vi "Set dts in Channel Groups.vi"(8 "error in":errorcluster, 9 "channel groups decimations":dbl[](array[numeric]), 11 "File Log Spec in":T1 {"File Node Ref" format="%.0x"}) -> (0 "error out":errorcluster, 3 "File Log Spec out":T1 {"File Node Ref" format="%.0x"})   [LabVIEW 2027, in "Embedded Data Logger Engine.lvlib"]
uses:
  Engine/Embedded Data Logger Engine.lvlib
  Engine/File Logging Specification.ctl
  Engine/Group Logging Specification.ctl
  Engine/Group Buffer Data.ctl
  Engine/Property Specification.ctl
  <vilib>/NI VeriStand/Custom Device API/Custom Device Item Ref.ctl
  Shared/Segment Files By.ctl
  Engine/Logging State.ctl
  <vilib>/NI VeriStand/Custom Device API/Custom Device API.lvlib
  Shared/Embedded Data Logger Shared.lvlib
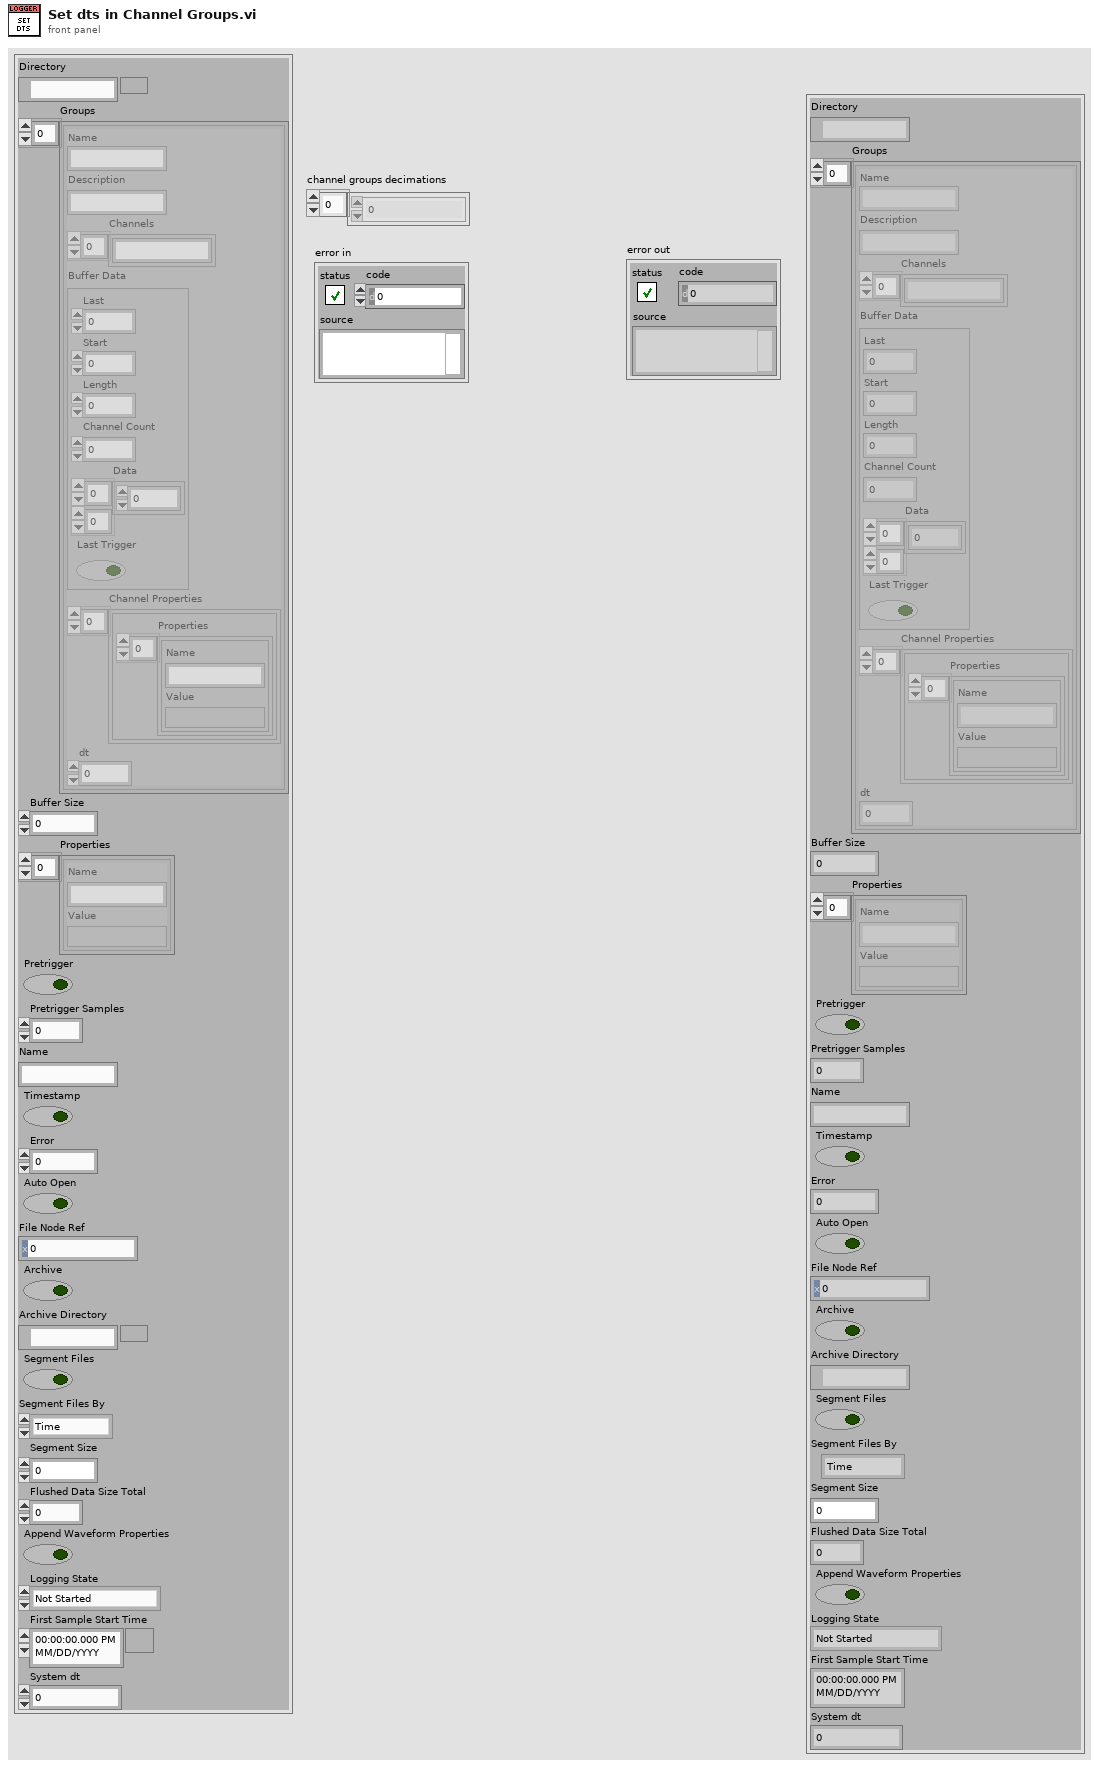
[diagram p1: front panel]
types:
  T1 = typedef "Embedded Data Logger Engine.lvlib/File Logging Specification.ctl" = cluster{"Directory":path, "Groups":T2[], "Buffer Size":i32, "Properties":T4[], "Pretrigger":bool, "Pretrigger Samples":i32, "Name":string, "Timestamp":bool, "Error":i32, "Auto Open":bool, "File Node Ref":T5, "Archive":bool, "Archive Directory":path, "Segment Files":bool, "Segment Files By":T6, "Segment Size":u32, "Flushed Data Size Total":u32, "Append Waveform Properties":bool, "Logging State":T7, "First Sample Start Time":timestamp, "System dt":dbl}
  T2 = typedef "Embedded Data Logger Engine.lvlib/Group Logging Specification.ctl" = cluster{"Name":string, "Description":string, "Channels":string[], "Buffer Data":T3, "Channel Properties":cluster{"Properties":T4[]}[], "dt":dbl}
  T3 = typedef "Embedded Data Logger Engine.lvlib/Group Buffer Data.ctl" = cluster{"Last":i32, "Start":i32, "Length":i32, "Channel Count":i32, "Data":dbl[][], "Last Trigger":bool}
  T4 = typedef "Embedded Data Logger Engine.lvlib/Property Specification.ctl" = cluster{"Name":string, "Value":variant}
  T5 = typedef "Custom Device API.lvlib/Custom Device Item Ref.ctl" = u64
  T6 = typedef "Embedded Data Logger Shared.lvlib/Segment Files By.ctl" = enum16{"Time", "Size"}
  T7 = typedef "Embedded Data Logger Engine.lvlib/Logging State.ctl" = enum16{"Not Started", "Continous Logging", "Paused", "Discontinous Logging"}
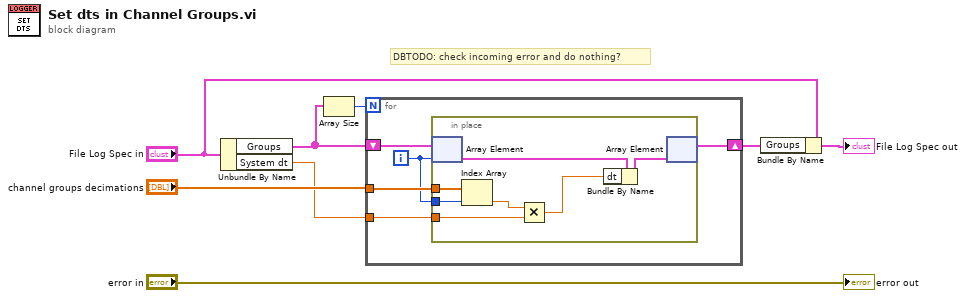
[diagram p0: block diagram]
diagram:
  # "DBTODO: check incoming error and do nothing?"
  n1 = Unbundle By Name("File Log Spec in") -> ("Groups"=w6:T2[], "System dt"=w1:dbl)
  n2 = Array Size(array=w6) -> (size(s)=w3:i32)
  n3 = for {
    N: w3 -> [_]
    shift-right: [w12] -> w7
    shift-left: w6 -> [w13]
    tunnel: "channel groups decimations" -> [w11]
    tunnel: w1 -> [w9]
    i -> [w10]
    n4 = in-place {
      in-place-border: w11 -> [w18]
      in-place-border: w10 -> [w17]
      in-place-border: w9 -> [w15]
      n5 = in-place-array #1(w13, w10) -> (w19:T2)
      n6 = Index Array(array=w18, index=w17) -> (element=w16:dbl)
      n7 = Multiply(x=w16, y=w15) -> (x*y=w14:dbl)
      n8 = Bundle By Name(cluster=w19, "dt"=w14) -> (w20:T2)
      n9 = in-place-array #1(w20) -> (w12:T2[])  [unwired: 1 out]
    }
  }
  n10 = Bundle By Name(cluster="File Log Spec in", "Groups"=w7) -> (→"File Log Spec out":T1)
  "error out" <- "error in"
